vi "Add to Parent.vi"(4 "Insertion Index":i32=-1, 6 "Unique ID":string, 7 "Parent ID":string, 8 "error in (no error)":errorcluster, 11 "Linked List in":refnum<class "Linked List.lvclass">) -> (0 "error out":errorcluster, 3 "Linked List out":refnum<class "Linked List.lvclass">)   [LabVIEW 2020, in "Linked Lists.lvlib" / "Linked List.lvclass"]
uses:
  <vilib>/gpm_packages/@cs/linked-list/Source/Linked List/Linked List/Linked List.lvclass
  <vilib>/gpm_packages/@cs/linked-list/Source/Linked List/Linked List Definition/Linked List Definition.lvclass
  <vilib>/gpm_packages/@cs/linked-list/Source/Linked List/Linked List/Linked List.lvclass/Linked List.ctl
  <vilib>/gpm_packages/@cs/lookup-table/Source/LookupTable/LookupTable.lvclass/LookupTable.ctl
  beab1386-fb03-4602-991d-c6dd99164584.vi
  9234b839-9e59-4810-9b93-2cc1a6eba5e0.vi
  <vilib>/gpm_packages/@cs/lookup-table/Source/LookupTable/Read Table Reference.vi
  beab1386-fb03-4602-991d-c6dd99164584.vi/2f5ce3b6-3f96-482a-b17f-d3a7e3a1cd87.vi
  9234b839-9e59-4810-9b93-2cc1a6eba5e0.vi/f20f29eb-a859-40ae-acdf-5e39be610159.vi
  <vilib>/gpm_packages/@cs/lookup-table/Source/LookupTable/LookupTable.lvclass
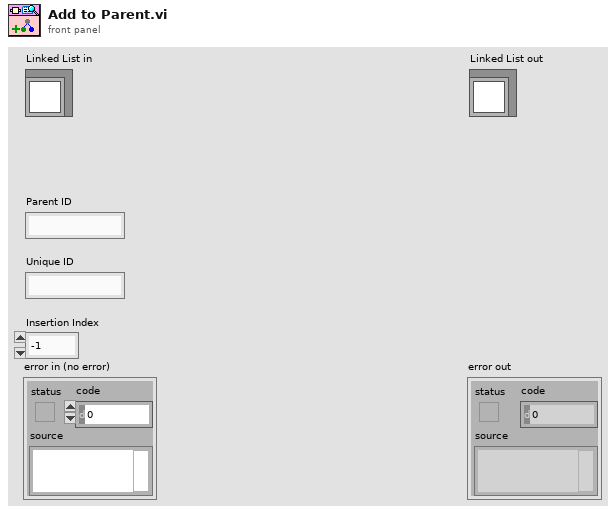
[diagram p1: front panel]
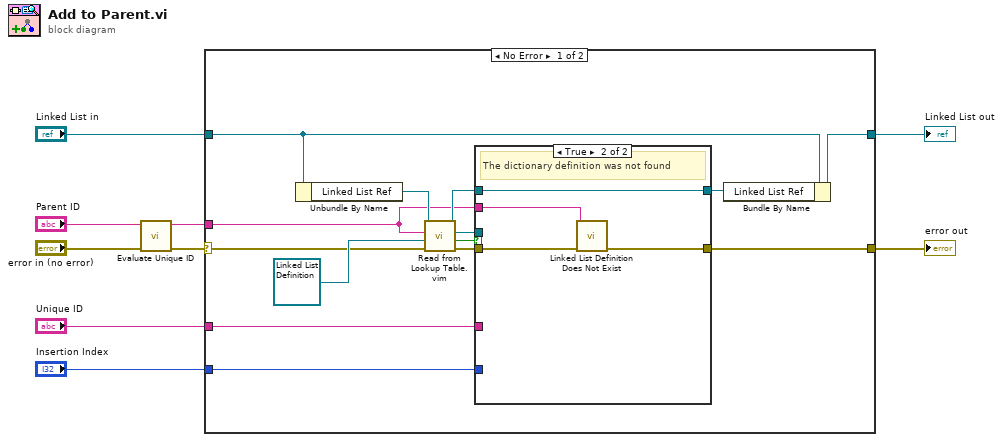
[diagram p0: block diagram]
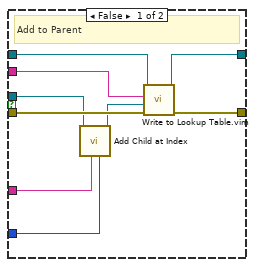
[diagram p2: hidden frame]
diagram:
  n1 = call <vilib>:"Evaluate Unique ID.vi"("error in (no error)"="error in (no error)", "Unique ID"="Parent ID") -> ("error out"=w6:errorcluster, "Unique ID Out"=w4:string)  [unwired: 8 in]
  n2 = case shown="No Error" w6 {
    selector: w6 -> [w14 w37]
    tunnel: [w15 w38] -> w7
    tunnel: "Linked List in" -> [w16 w38]
    tunnel: w4 -> [w13 _]
    tunnel: [w12 w37] -> w3
    tunnel: "Unique ID" -> [w11 _]
    tunnel: "Insertion Index" -> [w10 _]
    frame No Error {
      n3 = Unbundle By Name(w16) -> ("Linked List Ref"=w23:refnum<data-value>)
      n4 = call "Read from Lookup Table.vim"("error in (no error)"=w14, "Type"=refnum<class "Linked List Definition.lvclass"> refnum ("Linked List.lvlib:Linked List Definition.lvclass"), "Item Name"=w13, "LookupTable Reference"=w23) -> ("error out"=w18:errorcluster, "Not Found?"=w21:bool, "Value"=w19:refnum<class "Linked List Definition.lvclass">, "LookupTable Reference Out"=w20:refnum<data-value>)  [unwired: 4 in]
      n5 = case shown="True" w21 {
        tunnel: w20 -> [w30 w33]
        tunnel: w19 -> [w27 _]
        tunnel: [w31 w35] -> w12
        tunnel: w18 -> [w32 w36]
        tunnel: w13 -> [w29 w34]
        tunnel: w11 -> [w25 _]
        tunnel: [w28 w33] -> w17
        tunnel: w10 -> [w24 _]
        frame False {
          # "Add to Parent"
          n6 = call <vilib>:"Add Child at Index.vi"("Insertion Index"=w24, "Unique ID"=w25, "Linked List Definition in"=w27) -> ("Linked List Definition out"=w26:refnum<class "Linked List Definition.lvclass">)  [unwired: 8 in]
          n7 = call "Write to Lookup Table.vim"("error in (no error)"=w32, "Item"=w26, "Item Name"=w29, "LookupTable Reference"=w30) -> ("error out"=w31:errorcluster, "LookupTable Reference Out"=w28:refnum<data-value>)  [unwired: 5 in, 1 out]
        }
        frame True {
          # "The dictionary definition was not found"
          n8 = call <vilib>:"Linked List Definition Does Not Exist.vi"("Error In"=w36, "Unique ID"=w34) -> ("Error Out"=w35:errorcluster)  [unwired: 9 in]
        }
      }
      n9 = Bundle By Name(cluster=w16, "Linked List Ref"=w17) -> (w15:refnum<class "Linked List.lvclass">)
    }
    frame Error {
    }
  }
  "error out" <- w3
  "Linked List out" <- w7
